vi "RSNRPZ Get Sensor Info.vi"(8 "error in (no error)":errorcluster, 11 "Index (1)":i32=1 caption="Index (0)") -> (0 "error out":errorcluster, 1 "Sensor Type":string, 2 "Sensor Name":string, 4 "Sensor Serial Number":string)   [LabVIEW 2010]
doc: "This VI returns the name/descriptor of a connected sensor.\n\nIndex is  1...n   where 'n' is the number of connected sensors. \n'n' is evaluated by a call to rsnrpz_GetSensorCount() \n                                           \nThe char arrays pointed to by pszSensorName, pszSensorType and pszSensorSerial should provide room for 128 characters."
uses:
  rsnrpz_32.dll
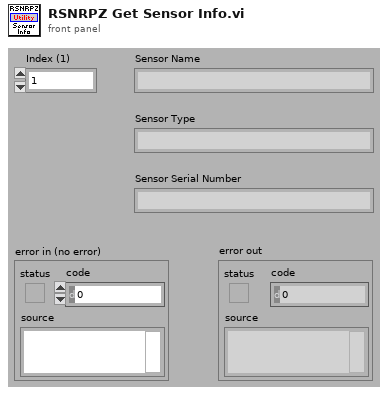
[diagram p1: front panel]
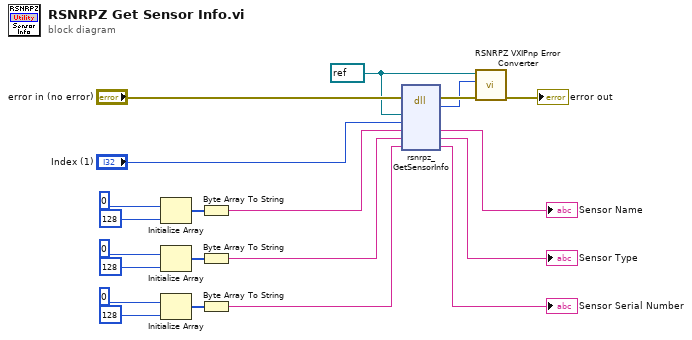
[diagram p0: block diagram]
diagram:
  w2 = refnum<visa-resource-name> refnum ("VISA session")
  n1 = Initialize Array(u8 0, 128) -> (w19:u8[])
  n2 = Initialize Array(u8 0, 128) -> (w16:u8[])
  n3 = Initialize Array(u8 0, 128) -> (w13:u8[])
  n4 = Byte Array To String(unsigned byte array=w19) -> (string=w11:string)
  n5 = Byte Array To String(unsigned byte array=w16) -> (string=w9:string)
  n6 = Byte Array To String(unsigned byte array=w13) -> (string=w7:string)
  n7 = dll-call lib="rsnrpz_32.dll" fn="rsnrpz_GetSensorInfo"(error in="error in (no error)", "Instrument Handle"=w2, "Channel"="Index (1)", "Sensor Name"=w11, "Sensor Type"=w9, "Sensor Serial"=w7) -> (error out=w4:errorcluster, "Status"=w1:i32, "Sensor Name"=→"Sensor Name":string, "Sensor Type"=→"Sensor Type":string, "Sensor Serial"=→"Sensor Serial Number":string)  [unwired: 4 in, 1 out]
  n8 = call <instrlib>:"RSNRPZ VXIPnp Error Converter.vi"("error in"=w4, "VXIPnp error code"=w1, "VISA session"=w2) -> ("error out"=→"error out":errorcluster)  [unwired: 7 in, 1 out]
